vi "Query Calibration Time Temperature.vi"(0 "VISA resource name":refnum<visa-resource-name>, 5 "Calibration Mode  (0: Time All)":i32(ring) items=["Time All", "Time Level", "Time Local", "Time Bandwidth", "Temperature All", "Temperature Level", "Temperature Local", "Temperature Bandwidth"], 11 "error in (no error)":errorcluster) -> (4 "VISA resource name out":refnum<visa-resource-name>, 6 "Time":i32, 10 "Temperature":dbl, 15 "error out":errorcluster)   [LabVIEW 2020, in "Anritsu Signal Analyzer Series.lvlib"]
doc: "Queries the time elapsed since the last All Calibration Time Command.\nQueries the time elapsed since the last Bandwidth Calibration.\nQueries the time elapsed since the last Local Leak calibration.\nQueries the time elapsed since the last Level Calibration."
uses:
  Anritsu Signal Analyzer Series.lvlib
panel:
  # "S or minutes"
  # "Celsius"
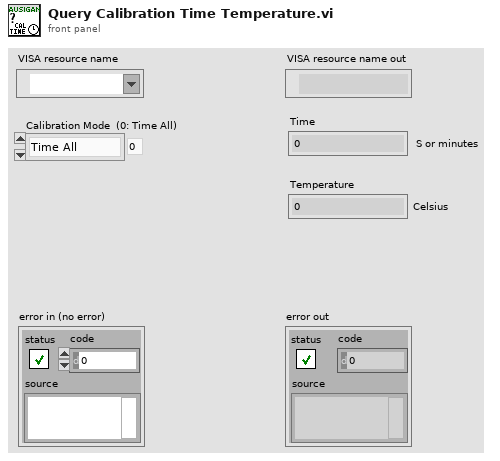
[diagram p1: front panel]
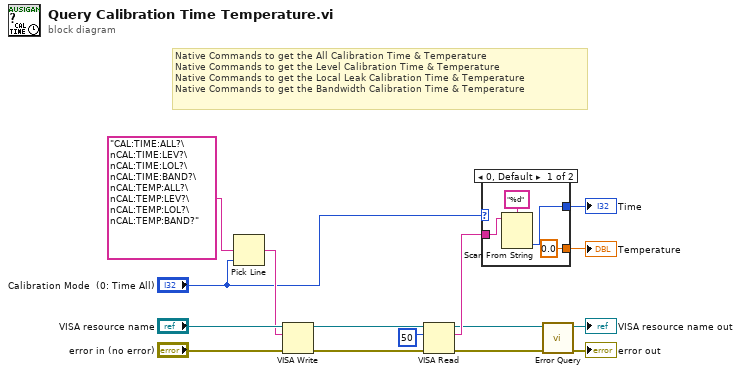
[diagram p0: block diagram]
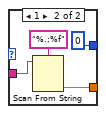
[diagram p2: hidden frame]
diagram:
  # "Native Commands to get the All Calibration Time & Temperature\nNative Commands to get the Level Calibration Time & Temperature\nNative Commands to get the Local Leak Calibration Time & Temperature\nNative Commands to get the Bandwidth Calibration Time & Temperature"
  n1 = Pick Line(multi-line string="CAL:TIME:ALL?\nCAL:TIME:LEV?\nCAL:TIME:LOL?\nCAL:TIME:BAND?\nCAL:TEMP:ALL?\nCAL:TEMP:LEV?\nCAL:TEMP:LOL?\nCAL:TEMP:BAND?" ("_Command"), line index="Calibration Mode  (0: Time All)") -> (output string=w3:string)  [unwired: 1 in]
  n2 = VISA Write(VISA resource name="VISA resource name", write buffer=w3, error in (no error)="error in (no error)") -> (VISA resource name out=w7:refnum<visa-resource-name>, error out=w8:errorcluster)  [unwired: 1 out]
  n3 = VISA Read(VISA resource name=w7, byte count=u32 50 ("byte count (0)"), error in (no error)=w8) -> (VISA resource name out=w5:refnum<visa-resource-name>, read buffer=w10:string, error out=w6:errorcluster)  [unwired: 1 out]
  n4 = case shown="0, Default" "Calibration Mode  (0: Time All)" {
    tunnel: [w19 0] -> w13
    tunnel: w10 -> [w17 w22]
    tunnel: [0.0 w20] -> w1
    frame 0, Default {
      n5 = Scan From String(format string="%d" ("Format String"), input string=w17) -> (output 1=w19:i32)  [unwired: 3 in, 3 out]
    }
    frame 1 {
      n6 = Scan From String(format string="%.;%f" ("Format String"), input string=w22) -> (output 1=w20:dbl)  [unwired: 3 in, 3 out]
    }
  }
  "Time" <- w13
  "Temperature" <- w1
  n7 = call "Error Query.vi"("error in (no error)"=w6, "VISA resource name"=w5) -> ("error out"=→"error out":errorcluster, "VISA resource name out"=→"VISA resource name out":refnum<visa-resource-name>)  [unwired: 6 in, 2 out]
